vi "Get cif_manager_ClockStatusArray.vi"(8 "error in (no error)":errorcluster, 11 "gRPCid":T1) -> (0 "error out":errorcluster, 2 "package_templatemessage":T2, 3 "gRPCid out":T1)   [LabVIEW 2021, in "CIF_Manager_server.lvlib"]
uses:
  CIF_Manager_server.lvlib
  cif_manager_ClockStatusArray.ctl
  cif_manager_ClockStatus.ctl
  cif_manager_ClockConversion.ctl
  cif_manager_TimePair.ctl
  <vilib>/gRPC/LabVIEW gRPC Library/Shared/grpcId.ctl
  cif_manager_ClockStatusArray_Flat.ctl
  cif_manager_ClockStatus_Flat.ctl
  cif_manager_ClockConversion_Flat.ctl
  cif_manager_TimePair_Flat.ctl
  2ed25e12-861d-4677-8ead-ace2906b2041.vi
  <vilib>/gRPC/LabVIEW gRPC Library/Shared/TranslateGrpcError.vi
  FlatToRichcif_manager_ClockStatus.vi
  FlatToRichcif_manager_ClockConversion.vi
  FlatToRichcif_manager_TimePair.vi
  <vilib>/gRPC/LabVIEW gRPC Library/Server API/Server/Get Server DLL Path.vi
  <vilib>/Utility/error.llb/Error Cluster From Error Code.vi
  <vilib>/gRPC/LabVIEW gRPC Library/grpc-lvsupport-release.lvlib
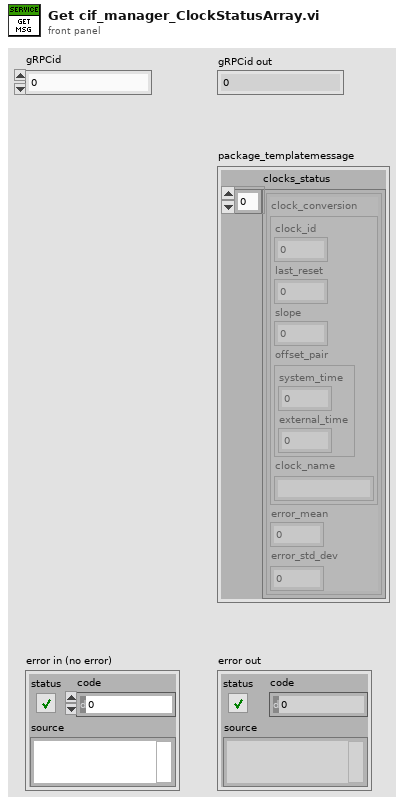
[diagram p1: front panel]
types:
  T1 = typedef "grpc-lvsupport-release.lvlib/grpcId.ctl" = u64
  T2 = typedef "CIF_Manager_server.lvlib/cif_manager_ClockStatusArray.ctl" = cluster{"clocks_status":T3[]}
  T3 = typedef "CIF_Manager_server.lvlib/cif_manager_ClockStatus.ctl" = cluster{"clock_conversion":T4, "error_mean":i64, "error_std_dev":i64}
  T4 = typedef "CIF_Manager_server.lvlib/cif_manager_ClockConversion.ctl" = cluster{"clock_id":u32, "last_reset":i64, "slope":dbl, "offset_pair":T5, "clock_name":string}
  T5 = typedef "CIF_Manager_server.lvlib/cif_manager_TimePair.ctl" = cluster{"system_time":i64, "external_time":i64}
  T6 = typedef "CIF_Manager_server.lvlib/cif_manager_ClockStatusArray_Flat.ctl" = cluster{"clocks_status":T7[]}
  T7 = typedef "CIF_Manager_server.lvlib/cif_manager_ClockStatus_Flat.ctl" = cluster{"clock_conversion":T8, "error_mean":i64, "error_std_dev":i64}
  T8 = typedef "CIF_Manager_server.lvlib/cif_manager_ClockConversion_Flat.ctl" = cluster{"clock_id":u32, "last_reset":i64, "slope":dbl, "offset_pair":T9, "clock_name":string}
  T9 = typedef "CIF_Manager_server.lvlib/cif_manager_TimePair_Flat.ctl" = cluster{"system_time":i64, "external_time":i64}
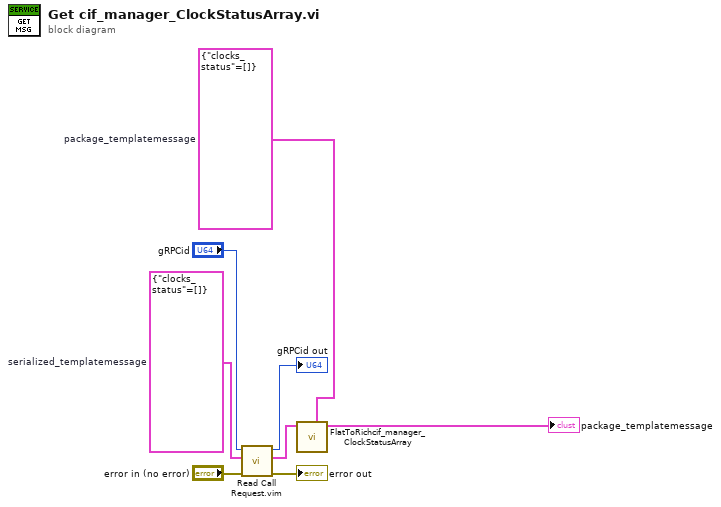
[diagram p0: block diagram]
diagram:
  w6 = T6 {"clocks_status"=[]}  # serialized_templatemessage
  w5 = T2 {"clocks_status"=[]}  # package_templatemessage
  n1 = call "Read Call Request.vim"("error in"="error in (no error)", "Request Type"=w6, "gRPCid in"="gRPCid") -> ("error out"=→"error out":errorcluster, "Request Data"=w4:T6, "gRPCid out"=→"gRPCid out":T1)  [unwired: 6 in]
  n2 = call "FlatToRichcif_manager_ClockStatusArray.vi"("OutputClusterType"=w5, "InputCluster"=w4) -> ("OutputCluster"=→"package_templatemessage":T2)  [unwired: 9 in]
